vi "HVIL.vi"(8 "error in":errorcluster caption="错误输入", 11 "Channel":u16=81 format="%.0x") -> (0 "error out":errorcluster caption="错误输出", 2 "频率/周期":u32, 3 "占空比":u32)   [LabVIEW 2020]
uses:
  <userlib>/PCANBasic/ctl/TPCANStatus.ctl
  <userlib>/PCANBasic/PCANBasic.lvlib
panel:
  out "TCANStatus 2":T1 items=["PCAN_ERROR_OK"=0, "PCAN_ERROR_XMTFULL"=1, "PCAN_ERROR_OVERRUN"=2, "PCAN_ERROR_BUSLIGHT"=4, "PCAN_ERROR_BUSHEAVY"=8, "PCAN_ERROR_BUSPASSIVE"=262144, "PCAN_ERROR_BUSOFF"=16, "PCAN_ERROR_QRCVEMPTY"=32, "PCAN_ERROR_QOVERRUN"=64, "PCAN_ERROR_QXMTFULL"=128, "PCAN_ERROR_REGTEST"=256, "PCAN_ERROR_NODRIVER"=512, "PCAN_ERROR_HWINUSE"=1024, "PCAN_ERROR_NETINUSE"=2048, "PCAN_ERROR_ILLHW"=5120, "PCAN_ERROR_ILLNET"=6144, "PCAN_ERROR_ILLCLIENT"=7168, "PCAN_ERROR_RESOURCE"=8192, "PCAN_ERROR_ILLPARAMTYPE"=16384, "PCAN_ERROR_ILLPARAMVAL"=32768, "PCAN_ERROR_UNKNOWN"=65536, "PCAN_ERROR_ILLDATA"=131072, "PCAN_ERROR_CAUTION"=33554432, "PCAN_ERROR_INITIALIZE"=67108864, "PCAN_ERROR_ILLOPERATION"=134217728]
  out "TCANStatus":T1 items=["PCAN_ERROR_OK"=0, "PCAN_ERROR_XMTFULL"=1, "PCAN_ERROR_OVERRUN"=2, "PCAN_ERROR_BUSLIGHT"=4, "PCAN_ERROR_BUSHEAVY"=8, "PCAN_ERROR_BUSPASSIVE"=262144, "PCAN_ERROR_BUSOFF"=16, "PCAN_ERROR_QRCVEMPTY"=32, "PCAN_ERROR_QOVERRUN"=64, "PCAN_ERROR_QXMTFULL"=128, "PCAN_ERROR_REGTEST"=256, "PCAN_ERROR_NODRIVER"=512, "PCAN_ERROR_HWINUSE"=1024, "PCAN_ERROR_NETINUSE"=2048, "PCAN_ERROR_ILLHW"=5120, "PCAN_ERROR_ILLNET"=6144, "PCAN_ERROR_ILLCLIENT"=7168, "PCAN_ERROR_RESOURCE"=8192, "PCAN_ERROR_ILLPARAMTYPE"=16384, "PCAN_ERROR_ILLPARAMVAL"=32768, "PCAN_ERROR_UNKNOWN"=65536, "PCAN_ERROR_ILLDATA"=131072, "PCAN_ERROR_CAUTION"=33554432, "PCAN_ERROR_INITIALIZE"=67108864, "PCAN_ERROR_ILLOPERATION"=134217728]
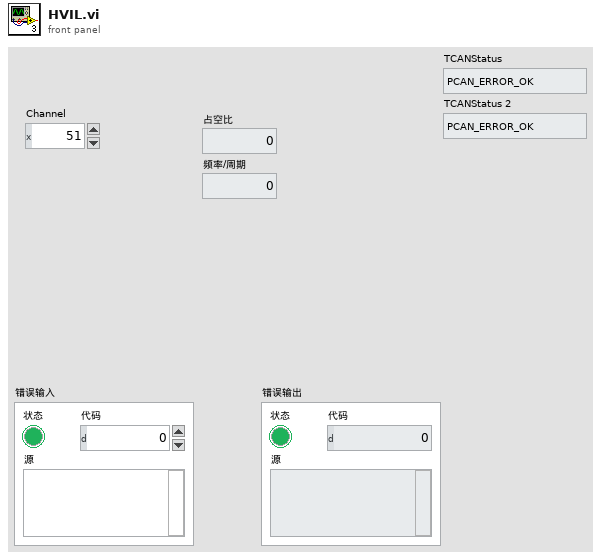
[diagram p1: front panel]
types:
  T1 = typedef "PCANBasic.lvlib/TPCANStatus.ctl" = u32
  T2 = typedef "PCANBasic.lvlib/TPCANMsgFD.ctl" = cluster{"ID":u32, "MSGTYPE":u8, "DLC":u8, "DATA":cluster{"[0]":u8, "[1]":u8, "[2]":u8, "[3]":u8, "[4]":u8, "[5]":u8, "[6]":u8, "[7]":u8, "[8]":u8, "[9]":u8, "[10]":u8, "[11]":u8, "[12]":u8, "[13]":u8, "[14]":u8, "[15]":u8, "[16]":u8, "[17]":u8, "[18]":u8, "[19]":u8, "[20]":u8, "[21]":u8, "[22]":u8, "[23]":u8, "[24]":u8, "[25]":u8, "[26]":u8, "[27]":u8, "[28]":u8, "[29]":u8, "[30]":u8, "[31]":u8, "[32]":u8, "[33]":u8, "[34]":u8, "[35]":u8, "[36]":u8, "[37]":u8, "[38]":u8, "[39]":u8, "[40]":u8, "[41]":u8, "[42]":u8, "[43]":u8, "[44]":u8, "[45]":u8, "[46]":u8, "[47]":u8, "[48]":u8, "[49]":u8, "[50]":u8, "[51]":u8, "[52]":u8, "[53]":u8, "[54]":u8, "[55]":u8, "[56]":u8, "[57]":u8, "[58]":u8, "[59]":u8, "[60]":u8, "[61]":u8, "[62]":u8, "[63]":u8}}
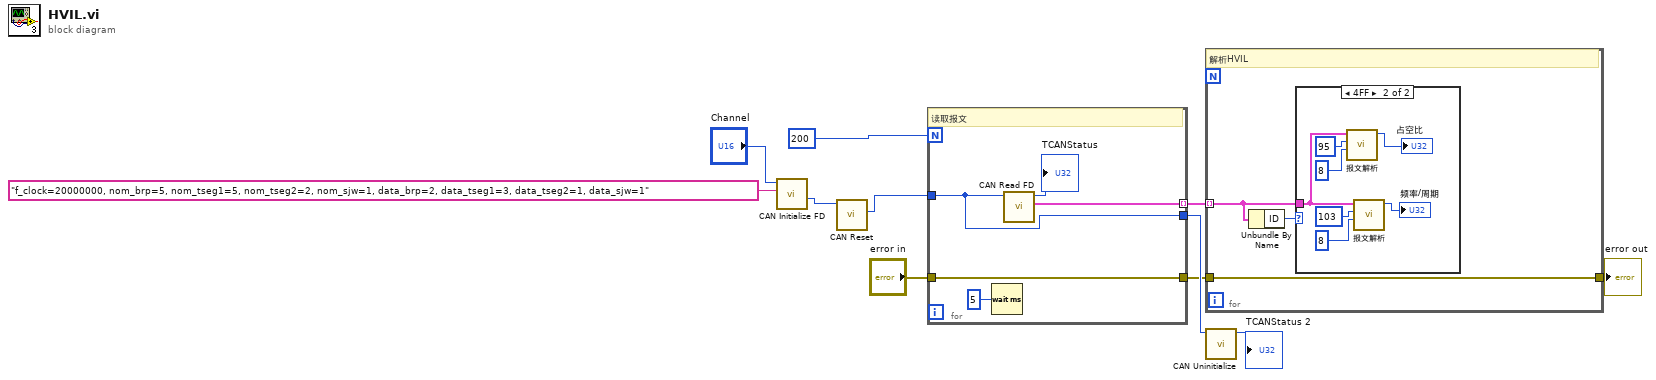
[diagram p0: block diagram]
diagram:
  n1 = call <userlib>:"CAN Initialize FD.vi"("BitrateFD"="f_clock=20000000, nom_brp=5, nom_tseg1=5, nom_tseg2=2, nom_sjw=1, data_brp=2, data_tseg1=3, data_tseg2=1, data_sjw=1", "Channel"="Channel") -> ("Channel out"=w3:u16)  [unwired: 6 in, 3 out]
  n2 = call <userlib>:"CAN Reset.vi"("Channel in"=w3) -> ("Channel out"=w2:u16)  [unwired: 8 in, 2 out]
  n3 = for {
    N: 200 -> [_]
    tunnel: [w15] -> w7 mode=indexing
    tunnel: w2 -> [w13]
    tunnel: [w13] -> w8
    tunnel: "error in" -> [w14]
    tunnel: [w14] -> w5
    # "读取报文"
    n4 = Wait (ms)(milliseconds to wait=u32 5 ("等待时间（毫秒）")) -> ()  [unwired: 1 out]
    n5 = call <userlib>:"CAN Read FD.vi"("Channel"=w13) -> ("MessageBuffer out"=w15:T2, "TCANStatus"=→"TCANStatus":T1)  [unwired: 7 in, 2 out]
  }
  n6 = for {
    tunnel: w7 -> [w18] mode=indexing
    tunnel: w5 -> [w17]
    tunnel: [w17] -> w4
    # "解析HVIL"
    n7 = Unbundle By Name(w18) -> ("ID"=w19:u32)
    n8 = case shown="4FF" w19 {
      tunnel: w18 -> [_ w24]
      frame 0, Default {
      }
      frame 1279 {
        n9 = call "报文解析.vi"("长度"=8, "起始位"=95, "MessageBuffer in"=w24) -> ("数字"=→"占空比":u32)  [unwired: 8 in]
        n10 = call "报文解析.vi"("长度"=8, "起始位"=103, "MessageBuffer in"=w24) -> ("数字"=→"频率/周期":u32)  [unwired: 8 in]
      }
    }
  }
  "error out" <- w4
  n11 = call <userlib>:"CAN Uninitialize.vi"("Channel"=w8) -> ("TCANStatus"=→"TCANStatus 2":T1)  [unwired: 9 in, 1 out]
